vi "CW Waveform Generator.vi"(6 "Word Gap":u8, 7 "Character Gap":u8, 8 "error in":errorcluster, 9 "Unit Speed (sec)":dbl, 10 "Plaintext Array":string[](array[string]), 11 "Plaintext to CW Map":map{string, bool[]}(c390)) -> (0 "error out":errorcluster, 3 "CW Waveform":waveform(dbl))   [LabVIEW 2026]
uses:
  <vilib>/Waveform/WDTOps.llb/WDT Append Waveforms DBL.vi
  <vilib>/measure/NI_MABase.lvlib
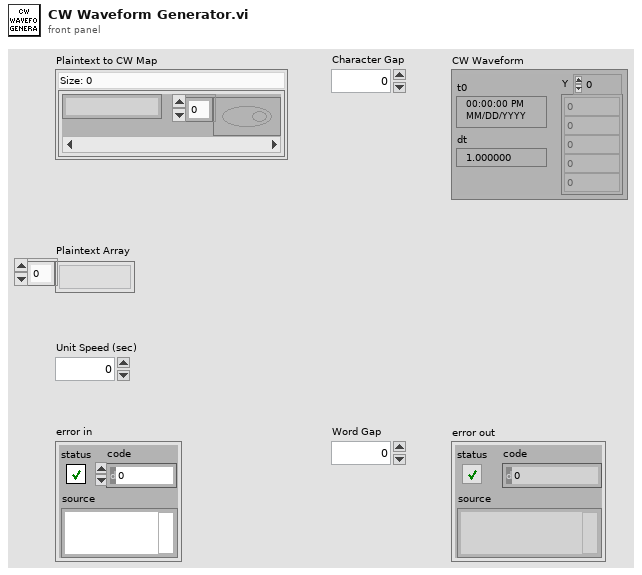
[diagram p1: front panel]
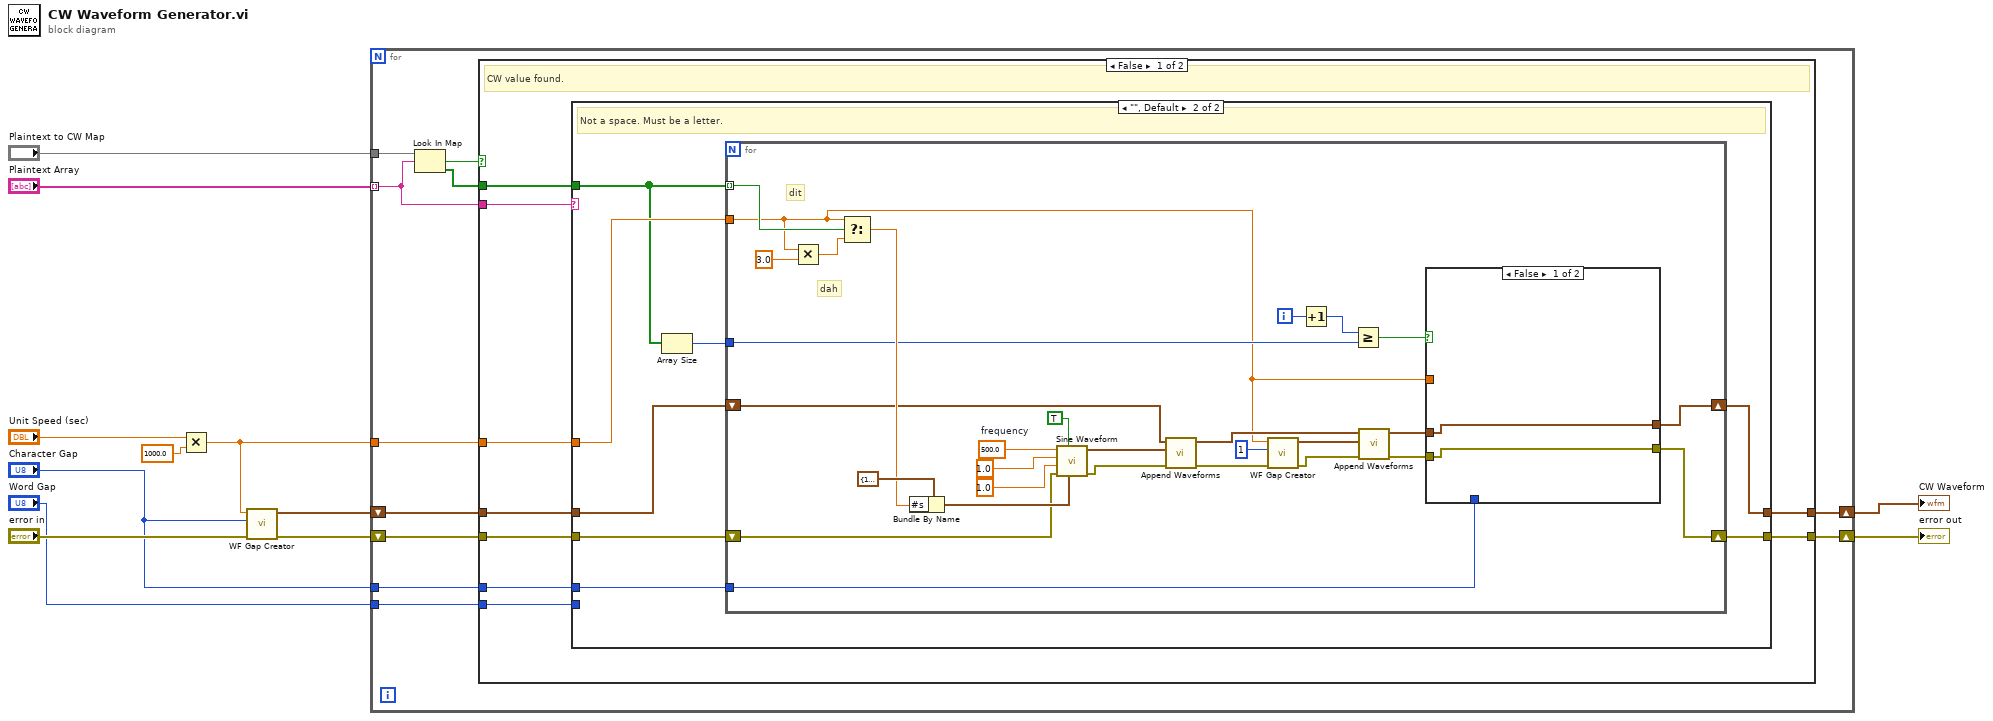
[diagram p0: block diagram]
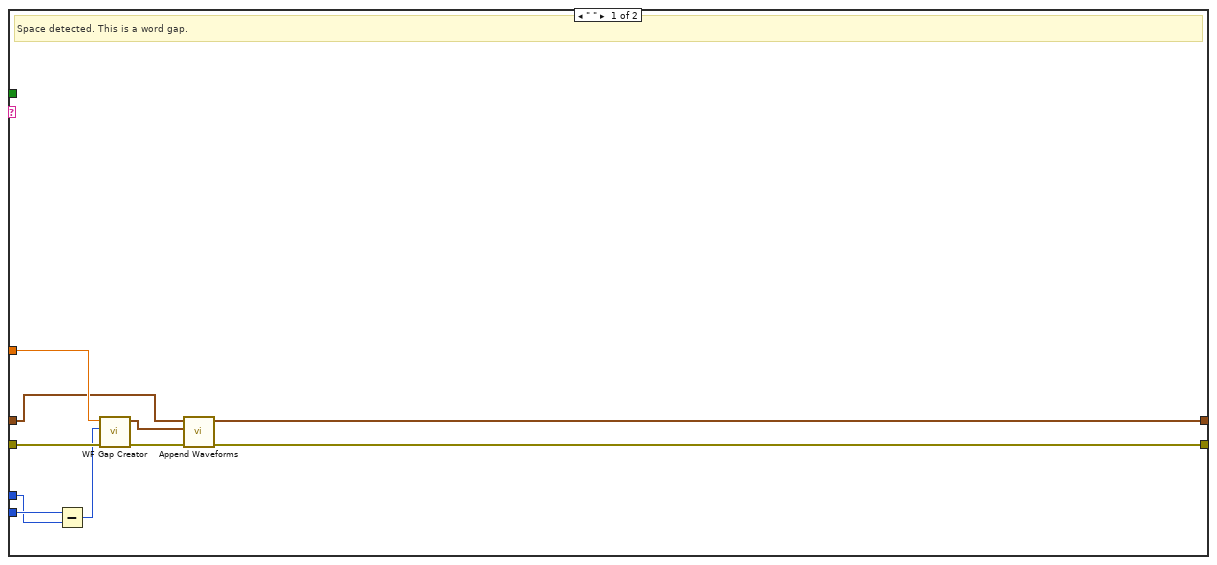
[diagram p2: hidden frame]
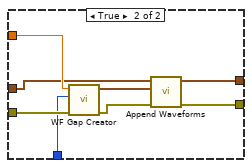
[diagram p3: hidden frame]
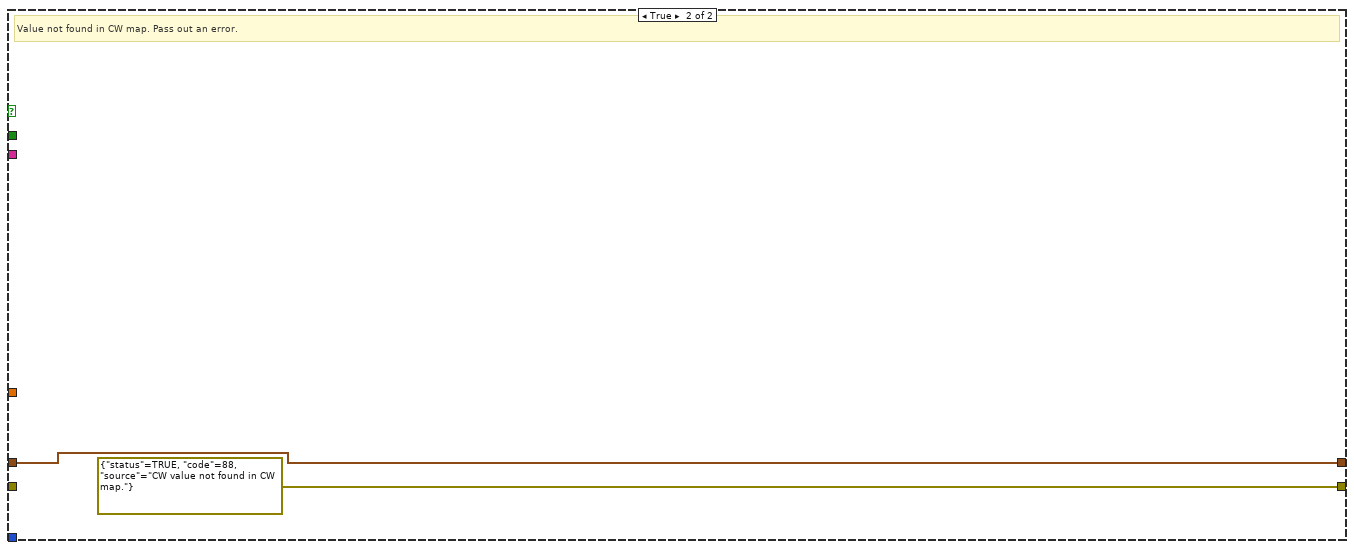
[diagram p4: hidden frame]
diagram:
  n1 = Multiply(x="Unit Speed (sec)", y=1000.0) -> (x*y=w5:dbl)
  n2 = call "WF Gap Creator.vi"("error in"="error in", "Character Gap"="Character Gap", "Unit Speed"=w5) -> ("error out"=w10:errorcluster, "waveform out"=w9:waveform(dbl))  [unwired: 7 in]
  n3 = for {
    tunnel: "Plaintext to CW Map" -> [w23]
    tunnel: "Plaintext Array" -> [w19] mode=indexing
    shift-right: [w21] -> w7
    shift-left: w10 -> [w20]
    tunnel: w5 -> [w18]
    tunnel: "Word Gap" -> [w17]
    tunnel: "Character Gap" -> [w16]
    shift-right: [w14] -> w1
    shift-left: w9 -> [w15]
    n4 = Look In Map(map=w23, key=w19) -> (key not found?=w22:bool, value=w13:bool[])  [unwired: 1 in]
    n5 = case shown="False" w22 {
      tunnel: [w26 errorcluster {"status"=TRUE, "code"=88, "source"="CW value not found in CW map."} ("error constant")] -> w21
      tunnel: w20 -> [w31 _]
      tunnel: w19 -> [w32 _]
      tunnel: w18 -> [w30 _]
      tunnel: w17 -> [w29 _]
      tunnel: w16 -> [w28 _]
      tunnel: w15 -> [w27 w90]
      tunnel: [w25 w90] -> w14
      tunnel: w13 -> [w24 _]
      frame False {
        # "CW value found."
        n6 = case shown="\"\", Default" w32 {
          tunnel: w31 -> [w42 w49]
          tunnel: w30 -> [w41 w50]
          tunnel: w29 -> [w40 _]
          tunnel: w28 -> [w39 w45]
          tunnel: w27 -> [w36 w48]
          tunnel: [w34 w43] -> w26
          tunnel: [w33 w44] -> w25
          tunnel: w24 -> [_ w47]
          frame " " {
            # "Decrement word gap by char gap since the last char dit/dah in a char has a char gap already appended."
            # "Space detected. This is a word gap."
            n7 = Subtract(x=w40, y=w39) -> (x-y=w38:u8)
            n8 = call "WF Gap Creator.vi"("error in"=w42, "Character Gap"=w38, "Unit Speed"=w41) -> ("error out"=w37:errorcluster, "waveform out"=w35:waveform(dbl))  [unwired: 7 in]
            n9 = call-poly <vilib>:"Append Waveforms.vi"("error in (no error)"=w37, "waveform B"=w35, "waveform A"=w36) -> ("error out"=w34:errorcluster, "waveform out"=w33:waveform(dbl))  [unwired: 7 in]
          }
          frame "", Default {
            # "Not a space. Must be a letter."
            n10 = Array Size(array=w47) -> (size(s)=w46:i32)
            n11 = for {
              tunnel: w47 -> [w79] mode=indexing
              tunnel: w50 -> [w55]
              tunnel: w46 -> [w58]
              tunnel: w45 -> [w54]
              shift-right: [w52] -> w44
              shift-left: w48 -> [w67]
              shift-right: [w51] -> w43
              shift-left: w49 -> [w69]
              i -> [w60]
              w74 = 500.0  # frequency
              # "dah"
              # "dit"
              n12 = Multiply(x=w55, y=3.0) -> (x*y=w78:dbl)
              n13 = Select(t=w55, s=w79, f=w78) -> (s? t:f=w75:dbl)
              n14 = Bundle By Name(cluster=cluster{"Fs":dbl, "#s":dbl} {"Fs"=1500.0, "#s"=1000.0} ("sampling info"), "#s"=w75) -> (w70:cluster{"Fs":dbl, "#s":dbl})
              n15 = call <vilib>:"Sine Waveform.vi"("sampling info"=w70, "reset signal"=TRUE, "error in (no error)"=w69, "phase"=1.0, "amplitude"=1.0, "frequency"=w74) -> ("error out"=w66:errorcluster, "signal out"=w68:waveform(dbl))  [unwired: 4 in]
              n16 = call-poly <vilib>:"Append Waveforms.vi"("error in (no error)"=w66, "waveform B"=w68, "waveform A"=w67) -> ("error out"=w65:errorcluster, "waveform out"=w63:waveform(dbl))  [unwired: 7 in]
              n17 = call "WF Gap Creator.vi"("error in"=w65, "Character Gap"=u8 1, "Unit Speed"=w55) -> ("error out"=w61:errorcluster, "waveform out"=w62:waveform(dbl))  [unwired: 7 in]
              n18 = Increment(x=w60) -> (x+1=w59:i32)
              n19 = Greater Or Equal?(x=w59, y=w58) -> (x >= y?=w57:bool)
              n20 = call-poly <vilib>:"Append Waveforms.vi"("error in (no error)"=w61, "waveform B"=w62, "waveform A"=w63) -> ("error out"=w56:errorcluster, "waveform out"=w53:waveform(dbl))  [unwired: 7 in]
              n21 = case shown="False" w57 {
                tunnel: w56 -> [w80 w89]
                tunnel: w55 -> [_ w88]
                tunnel: w54 -> [_ w87]
                tunnel: w53 -> [w81 w84]
                tunnel: [w81 w83] -> w52
                tunnel: [w80 w82] -> w51
                frame False {
                }
                frame True {
                  n22 = call "WF Gap Creator.vi"("error in"=w89, "Character Gap"=w87, "Unit Speed"=w88) -> ("error out"=w85:errorcluster, "waveform out"=w86:waveform(dbl))  [unwired: 7 in]
                  n23 = call-poly <vilib>:"Append Waveforms.vi"("error in (no error)"=w85, "waveform B"=w86, "waveform A"=w84) -> ("error out"=w82:errorcluster, "waveform out"=w83:waveform(dbl))  [unwired: 7 in]
                }
              }
            }
          }
        }
      }
      frame True {
        # "Value not found in CW map. Pass out an error."
      }
    }
  }
  "error out" <- w7
  "CW Waveform" <- w1
